vi "New from WAMP message.vi"(8 "error in (no error)":errorcluster, 11 "wamplv.lvlib:JSONMessage.lvclass":refnum<class "WampMessage JSON.lvclass">) -> (0 "error out":errorcluster, 1 "Error data (JSON)":T1={"Request ID"=0, "Message type that caused error"=enum."HELLO", "Error/Abort details (JSON)"={"Error URI"="", "Error Arguments"="", "Error ArgumentKw"="{}", "Error Details"="{}"}}, 2 "Request ID":u64, 3 "ErrorHandler JSON out":refnum<class "ErrorHandler JSON.lvclass">)   [LabVIEW 2020, in "wamplv.lvlib" / "ErrorHandler JSON.lvclass"]
uses:
  ErrorHandler JSON.lvclass
  SerialisedMessages/JSONMessage/WampMessage JSON.lvclass
  WAMP Client/API/TypeDefs/Error or abort detail (JSON).ctl
  wamplv.lvlib
  TypeDefs/WAMP Message Codes.ctl
  WAMP Client/Private/TypeDef/Error (JSON).ctl
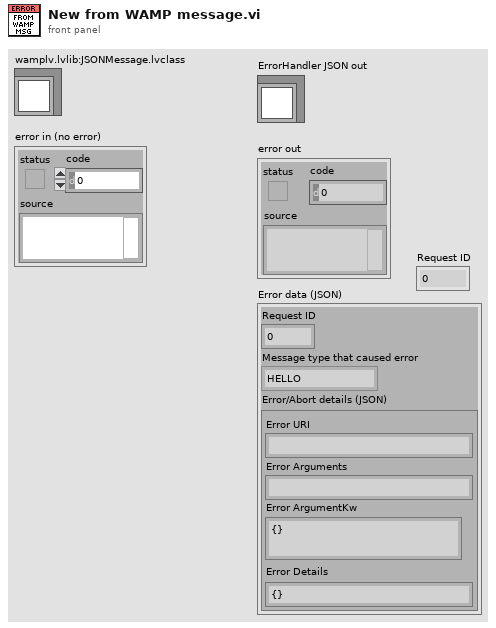
[diagram p1: front panel]
types:
  T1 = typedef "wamplv.lvlib/Error (JSON).ctl" = cluster{"Request ID":u64, "Message type that caused error":T2, "Error/Abort details (JSON)":T3}
  T2 = typedef "wamplv.lvlib/WAMP Message Codes.ctl" = enum8{"HELLO", "WELCOME", "CHALLENGE", "AUTHENTICATE", "ABORT", "GOODBYE", "ERROR", "PUBLISH", "PUBLISHED", "SUBSCRIBE", "SUBSCRIBED", "UNSUBSCRIBE", "UNSUBSCRIBED", "EVENT", "CALL", "RESULT", "REGISTER", "REGISTERED", "UNREGISTER", "UNREGISTERED", "INVOCATION", "YIELD"}
  T3 = typedef "wamplv.lvlib/Error or abort detail (JSON).ctl" = cluster{"Error URI":string, "Error Arguments":string, "Error ArgumentKw":string, "Error Details":string}
  T4 = typedef "wamplv.lvlib/Error (JSON).ctl" = cluster{"Request ID":u64, "Message type that caused error":T2, "Error/Abort details (JSON)":T5}
  T5 = typedef "wamplv.lvlib/Error or abort detail (JSON).ctl" = cluster{"Error URI":string, "Error Arguments":string, "Error ArgumentKw":string, "Error Details":string, "Associated LabVIEW Error":errorcluster}
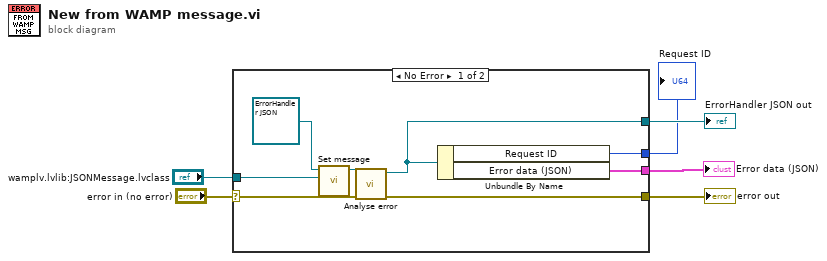
[diagram p0: block diagram]
diagram:
  n1 = case shown="No Error" "error in (no error)" {
    selector: "error in (no error)" -> [w11 w15]
    tunnel: [w10 w15] -> w5
    tunnel: "wamplv.lvlib:JSONMessage.lvclass" -> [w13 _]
    tunnel: [w9 _] -> w3
    tunnel: [w8 _] -> w2
    tunnel: [w7 _] -> w1
    frame No Error {
      n2 = call-dynamic "Set message.vi"("WampMessage JSON"=w13, "ErrorHandler JSON in"=refnum<class "ErrorHandler JSON.lvclass"> refnum ("wamplv.lvlib:ErrorHandler JSON.lvclass")) -> ("ErrorHandler JSON out"=w12:refnum<class "ErrorHandler JSON.lvclass">)  [unwired: 9 in]
      n3 = call-dynamic "Analyse error.vi"("error in (no error)"=w11, "ErrorHandler JSON in"=w12) -> ("error out"=w10:errorcluster, "ErrorHandler JSON out"=w9:refnum<class "ErrorHandler JSON.lvclass">)  [unwired: 8 in]
      n4 = Unbundle By Name(w9) -> ("Request ID"=w7:u64, "Error data (JSON)"=w8:T4)
    }
    frame Error {
    }
  }
  "error out" <- w5
  "ErrorHandler JSON out" <- w3
  "Error data (JSON)" <- w2
  "Request ID" <- w1
